vi "myRIO_BRig_FPGA_laserPulse__v2.vi"(0 "I_shutter":bool, 1 "I_peak":bool, 2 "count":u32, 3 "laser_Nshutter":u32=100, 4 "laser_Npeak":u32=100, 5 "laser_Nvalley":u32=100, 6 "I_laserEvent":bool, 8 "I_laser":bool) -> (14 "output_I_shutter":bool, 15 "output_I_peak":bool, 16 "output_count":u32, 17 "output_shutter":bool, 18 "output_led":bool, 19 "output_laser":bool)   [LabVIEW 2014]
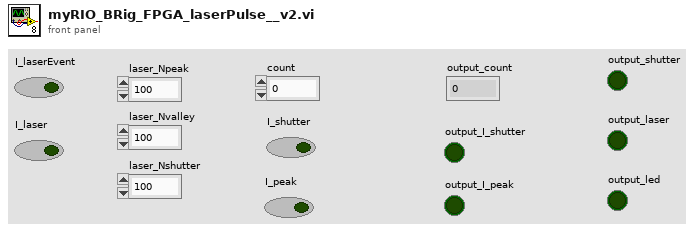
[diagram p1: front panel]
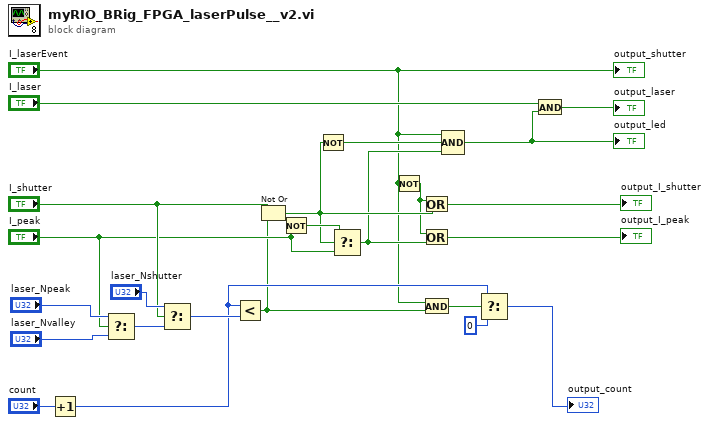
[diagram p0: block diagram]
diagram:
  n1 = Increment(x="count") -> (x+1=w18:u32)
  n2 = Select(t="laser_Npeak", s="I_peak", f="laser_Nvalley") -> (s? t:f=w22:u32)
  n3 = Select(t="laser_Nshutter", s="I_shutter", f=w22) -> (s? t:f=w19:u32)
  n4 = Less?(x=w18, y=w19) -> (x < y?=w5:bool)
  n5 = Not Or(1:w5, 2:"I_shutter") -> (0:w4:bool)
  n6 = Not(x="I_peak") -> (.not. x?=w10:bool)
  n7 = Not(x=w4) -> (.not. x?=w8:bool)
  n8 = Select(t=w10, s=w4, f="I_peak") -> (s? t:f=w3:bool)
  n9 = Not(x="I_laserEvent") -> (.not. x?=w2:bool)
  n10 = Or(x=w2, y=w4) -> (x .or. y?=→"output_I_shutter":bool)
  n11 = Or(x=w2, y=w3) -> (x .or. y?=→"output_I_peak":bool)
  n12 = And(x="I_laserEvent", y=w5) -> (x .and. y?=w6:bool)
  n13 = Compound Arithmetic op=AND("I_laserEvent", w8, w3) -> (w7:bool)
  "output_led" <- w7
  n14 = Select(t=w18, s=w6, f=u32 0) -> (s? t:f=→"output_count":u32)
  n15 = And(x="I_laser", y=w7) -> (x .and. y?=→"output_laser":bool)
  "output_shutter" <- "I_laserEvent"
